vi "Check.vi"(8 "error in (no error)":errorcluster) -> (0 "error out":errorcluster, 2 "Passed":bool)   [LabVIEW 2017, in "WebServiceImporter.lvlib" / "Main Panel.lvlib" / "Input Info.lvlib"]
uses:
  <vilib>/Platform/WebService/Main Panel/Pages/Input Info/Input Info.lvlib
  <vilib>/Platform/WebService/Main Panel/Events/Events.lvlib
  <vilib>/Platform/WebService/Main Panel/Pages/Input Info/Events/Events.lvlib
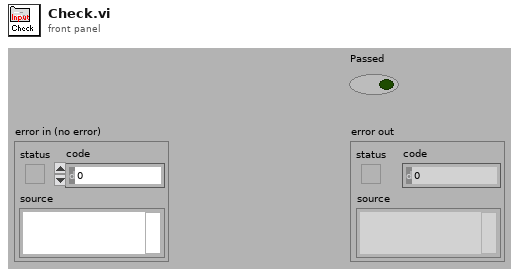
[diagram p1: front panel]
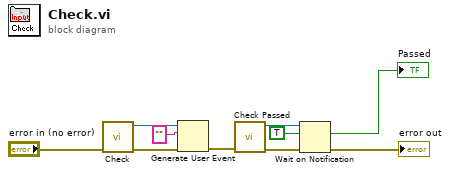
[diagram p0: block diagram]
diagram:
  n1 = call <vilib>:"Check.vi"("error in (no error)"="error in (no error)") -> ("error out"=w4:errorcluster, "user event (out)"=w7:refnum<user-event>)  [unwired: 9 in]
  n2 = Generate User Event(user event=w7, event data cluster="" ("event data"), error in=w4) -> (error out=w3:errorcluster)  [unwired: 1 in, 1 out]
  n3 = call <vilib>:"Check Passed.vi"("error in (no error)"=w3) -> ("error out"=w2:errorcluster, "notifier  (out)"=w8:refnum<notifier>)  [unwired: 9 in]
  n4 = Wait on Notification(notifier=w8, ignore previous (F)=TRUE, error in (no error)=w2) -> (notification=→"Passed":bool, error out=→"error out":errorcluster)  [unwired: 1 in, 2 out]
